vi "rampsStates(Final).vi"(6 "buttonsPushed?":bool, 7 "endGame?":bool, 8 "stage2Clear?":bool, 9 "motor2Stop":bool, 10 "motor1Stop":bool) -> (1 "motor2":bool, 2 "motor1":bool)   [LabVIEW 2017]
uses:
  rampsLogicStates.ctl
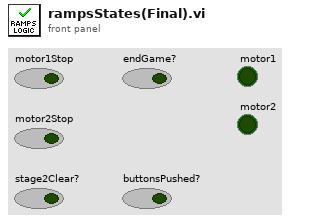
[diagram p1: front panel]
types:
  T1 = typedef "rampsLogicStates.ctl" = enum16{"endGame", "finish", "idle", "deploy"}
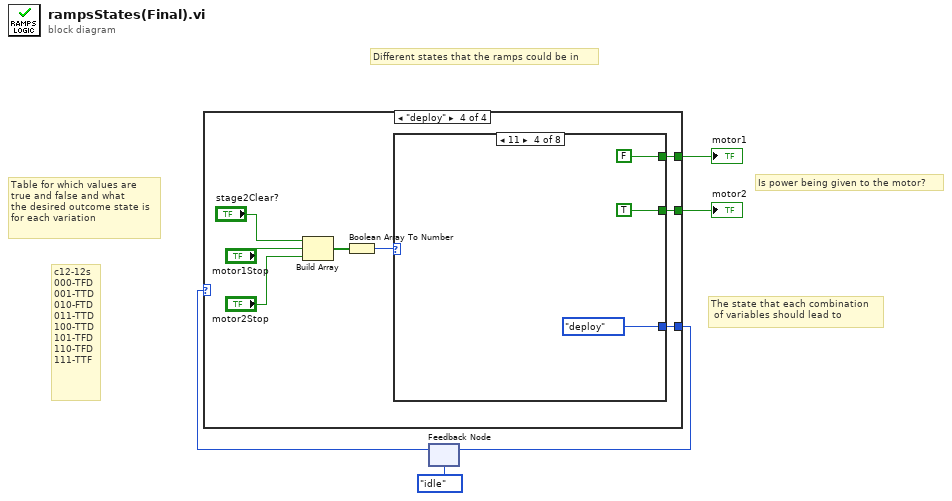
[diagram p0: block diagram]
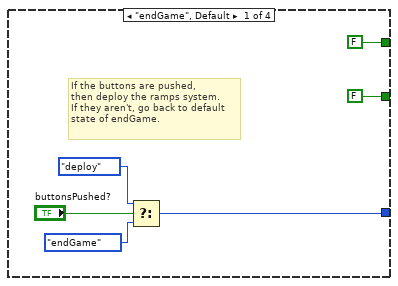
[diagram p2: hidden frame]
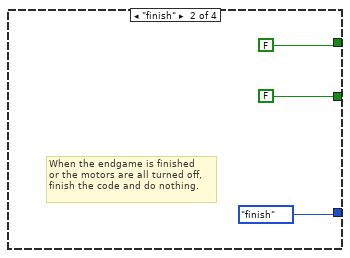
[diagram p3: hidden frame]
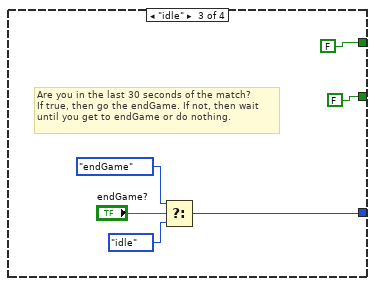
[diagram p4: hidden frame]
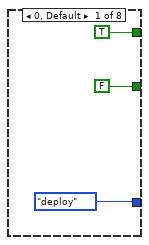
[diagram p5: hidden frame]
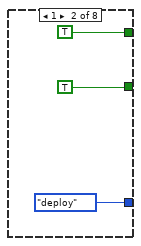
[diagram p6: hidden frame]
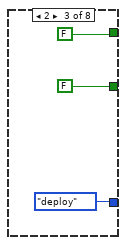
[diagram p7: hidden frame]
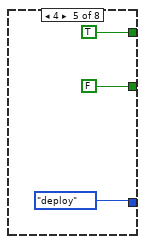
[diagram p8: hidden frame]
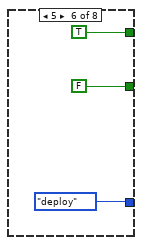
[diagram p9: hidden frame]
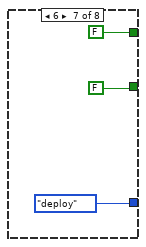
[diagram p10: hidden frame]
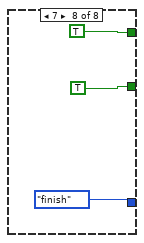
[diagram p11: hidden frame]
diagram:
  # "The state that each combination\n of variables should lead to"
  # "Is power being given to the motor?"
  # "Different states that the ramps could be in"
  # "Table for which values are\ntrue and false and what\nthe desired outcome state is\nfor each variation"
  # "c12-12s\n000-TFD\n001-TTD\n010-FTD\n011-TTD\n100-TTD\n101-TFD\n110-TFD\n111-TTF"
  n1 = feedback #1(rampsLogicStates."idle") -> (w2:T1)
  n2 = case shown="\"deploy\"" w2 {
    tunnel: [w8 rampsLogicStates."finish" w19 w21] -> w3
    tunnel: [FALSE FALSE FALSE w25] -> w4
    tunnel: [FALSE FALSE FALSE w26] -> w5
    frame "endGame", Default {
      # "If the buttons are pushed, \nthen deploy the ramps system.\nIf they aren't, go back to default\nstate of endGame."
      n3 = Select(t=rampsLogicStates."deploy", s="buttonsPushed?", f=rampsLogicStates."endGame") -> (s? t:f=w8:T1)
    }
    frame "finish" {
      # "When the endgame is finished\nor the motors are all turned off,\nfinish the code and do nothing."
    }
    frame "idle" {
      # "Are you in the last 30 seconds of the match?\nIf true, then go the endGame. If not, then wait\nuntil you get to endGame or do nothing."
      n4 = Select(t=rampsLogicStates."endGame", s="endGame?", f=rampsLogicStates."idle") -> (s? t:f=w19:T1)
    }
    frame "deploy" {
      n5 = Build Array("stage2Clear?", "motor1Stop", "motor2Stop") -> (w28:bool[])
      n6 = Boolean Array To Number(Boolean array=w28) -> (number=w27:u32)
      n7 = case shown="11" w27 {
        tunnel: [TRUE TRUE FALSE FALSE TRUE TRUE FALSE TRUE] -> w26
        tunnel: [FALSE TRUE FALSE TRUE FALSE FALSE FALSE TRUE] -> w25
        tunnel: [rampsLogicStates."deploy" rampsLogicStates."deploy" rampsLogicStates."deploy" rampsLogicStates."deploy" rampsLogicStates."deploy" rampsLogicStates."deploy" rampsLogicStates."deploy" rampsLogicStates."finish"] -> w21
        frame 0, Default {
        }
        frame 1 {
        }
        frame 2 {
        }
        frame 3 {
        }
        frame 4 {
        }
        frame 5 {
        }
        frame 6 {
        }
        frame 7 {
        }
      }
    }
  }
  "motor1" <- w5
  "motor2" <- w4
  n8 = feedback-in #1(w3) -> ()
